vi "get dt.vi"(11 "timing source in":refnum<class "TBM timing source.lvclass">) -> (2 "dt":u32=1, 3 "timing source out":refnum<class "TBM timing source.lvclass">)   [LabVIEW 2013, in "TBM timing source.lvclass"]
doc: "Returns the value of <b>dt</b> which is the number of ticks of the desired clock which should elapse between iterations. This behavior is generally the same as the behavior of the timed loop."
uses:
  TBM timing source.lvclass
  TBM timing source.lvclass/TBM timing source.ctl
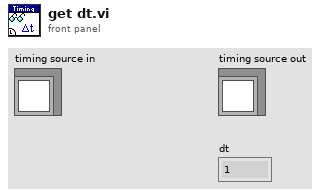
[diagram p1: front panel]
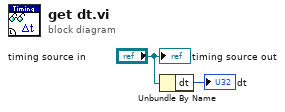
[diagram p0: block diagram]
diagram:
  n1 = Unbundle By Name("timing source in") -> ("dt"=→"dt":u32)
  "timing source out" <- "timing source in"
